vi "update.labels.request.vi"(8 "error in":errorcluster, 11 "Labels":string[](array[string])) -> (0 "error out":errorcluster, 1 "Request":string)   [LabVIEW 2020, in "asset.lvclass"]
uses:
  asset.lvclass
  fc7aacf3-d9fa-4911-86be-9d011dabdec1.vi
  <vilib>/JDP Science/JSONtext/Variant to JSON Text.vi
  <vilib>/JDP Science/JSONtext/LVClass Serializer/JSONtext LVClass Serializer.lvclass
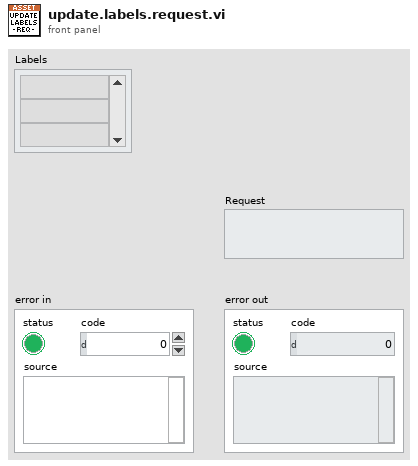
[diagram p1: front panel]
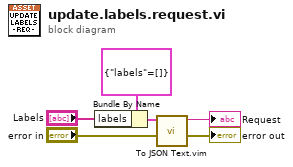
[diagram p0: block diagram]
diagram:
  n1 = Bundle By Name(cluster=cluster{"labels":string[]} {"labels"=[]}, "labels"="Labels") -> (w6:cluster{"labels":string[]})
  n2 = call "To JSON Text.vim"("error in (no error)"="error in", "Anything"=w6) -> ("error out"=→"error out":errorcluster, "<JSON>"=→"Request":string)  [unwired: 8 in]
